vi "Ctor.vi"(8 "error in (no error)":errorcluster, 11 "SerialConfigPanel in":refnum<class "SerialConfigPanel.lvclass">) -> (0 "error out":errorcluster, 3 "SerialConfigPanel out":refnum<class "SerialConfigPanel.lvclass">)   [LabVIEW 2020, in "LV-Term.lvlib" / "SerialConfigPanel.lvclass"]
uses:
  SerialConfigPanel.lvclass
  SerialConfigPanel.lvclass/SerialConfigPanel.ctl
  <vilib>/IlluminatedG/IG Serial Stream/Stream-Serial/Serial Client/Stop Bits.ctl
  <vilib>/IlluminatedG/IG Serial Stream/Stream-Serial/Serial Client/Serial Client.lvclass
  <vilib>/IlluminatedG/IG Serial Stream/Stream-Serial/Serial Client/Flow Control.ctl
  <vilib>/IlluminatedG/IG Serial Stream/Stream-Serial/Serial Client/Parity.ctl
  <vilib>/IlluminatedG/IG Serial Stream/Stream-Serial/Serial Client/Port Config.ctl
  Ref Data.ctl
  <vilib>/IlluminatedG/IG OOPanel/OOPanel/Panel/Panel.lvclass
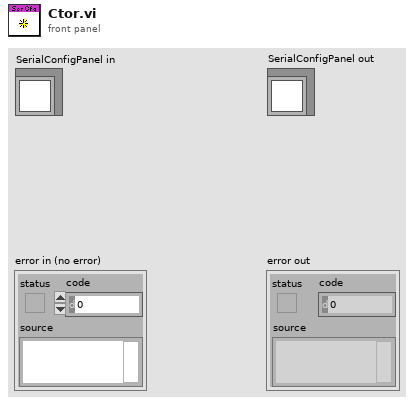
[diagram p1: front panel]
types:
  T1 = typedef "LV-Term.lvlib/SerialConfigPanel.lvclass/Ref Data.ctl" = cluster{"Port":refnum<visa-resource-name>, "Config":T2}
  T2 = typedef "Stream-Serial.lvlib/Serial Client.lvclass/Port Config.ctl" = cluster{"Baud (115200)":u32, "Data Bits (8)":u8, "Stop Bits (1)":T3, "Flow Control":T4, "Use LineTerm?":bool, "LineTerm (\\n)":string, "Timeout ms (10000)":i32, "Parity (None)":T5}
  T3 = typedef "Stream-Serial.lvlib/Serial Client.lvclass/Stop Bits.ctl" = u16
  T4 = typedef "Stream-Serial.lvlib/Serial Client.lvclass/Flow Control.ctl" = u16
  T5 = typedef "Stream-Serial.lvlib/Serial Client.lvclass/Parity.ctl" = enum16{"None", "Odd", "Even", "Mark", "Space"}
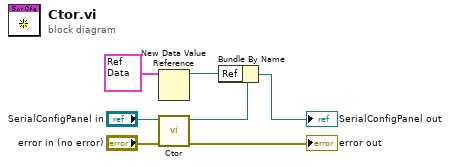
[diagram p0: block diagram]
diagram:
  n1 = New Data Value Reference(data value=T1 {"Port"="", "Config"={"Baud (115200)"=115200, "Data Bits (8)"=8, "Stop Bits (1)"=10, "Flow Control"=0, "Use LineTerm?"=FALSE, "LineTerm (\\n)"="\n", "Timeout ms (10000)"=10000, "Parity (None)"=enum."None"}} ("Ref Data")) -> (data value reference=w5:refnum<data-value>)  [unwired: 1 in, 1 out]
  n2 = call-parent "Ctor.vi"("error in (no error)"="error in (no error)", "Panel in"="SerialConfigPanel in") -> ("error out"=→"error out":errorcluster, "Panel out"=w1:refnum<class "SerialConfigPanel.lvclass">)  [unwired: 8 in]
  n3 = Bundle By Name(cluster=w1, "Ref"=w5) -> (→"SerialConfigPanel out":refnum<class "SerialConfigPanel.lvclass">)
